vi "Select HDF5 Dialog Core.vi"(0 "Initial File Path":path, 1 "Close HDF5 File?":bool, 2 "Item Filters":T4 {"Object Types (any)" items=["H5G_UNKNOWN"=-1, "H5G_GROUP"=0, "H5G_DATASET"=1, "H5G_TYPE"=2, "H5G_LINK"=3, "H5G_UDLINK"=4]}, 3 "File Browse Options":T7, 5 "HDF5 File Ref":T9, 7 "Initial Object Path":string, 9 "Path visible":bool=TRUE, 11 "error in":errorcluster, 12 "Operation Modes":cluster{"File":T1, "Object":T2}={"File"=enum."open or create", "Object"=enum."open or create"}, 13 "Window":T6={"Behavior"=enum."Modal", "Position"={"Left"=0, "Top"=0, "Right"=600, "Bottom"=400}, "Center"=TRUE, "Title"="Select an HDF5 Object"}) -> (4 "File Path out":path, 6 "HDF5 File Ref out":T9, 8 "Object Path out":string, 10 "OK?":bool, 14 "Object operation out":T8(ring), 15 "error out":errorcluster)   [LabVIEW 2017]
uses:
  <vilib>/UPVI/lvhdf5/library.llb/HDF5 Ref.ctl
  <vilib>/Utility/miscctls.llb/LVRectTypeDef.ctl
  <vilib>/UPVI/lvhdf5/group.llb/H5G_obj_t.ctl
  <vilib>/UPVI/lvhdf5/file.llb/LVH5F Operation.ctl
  <vilib>/UPVI/lvhdf5/dataset.llb/LVH5D Operation.ctl
  <vilib>/UPVI/lvhdf5/utility.llb/private/TreeIconsEnum.ctl
  <vilib>/UPVI/lvhdf5/object.llb/H5O_type_t.ctl
  <vilib>/UPVI/lvhdf5/identifier.llb/H5Iget_type.vi
panel:
  in  "File Path":path
  in  "Object Path":string
  in  "Cancel Button":bool
  in  "OK Button":bool
  in  "Attributes":i32(listbox)
  in  "Hierarchy":string(tree)
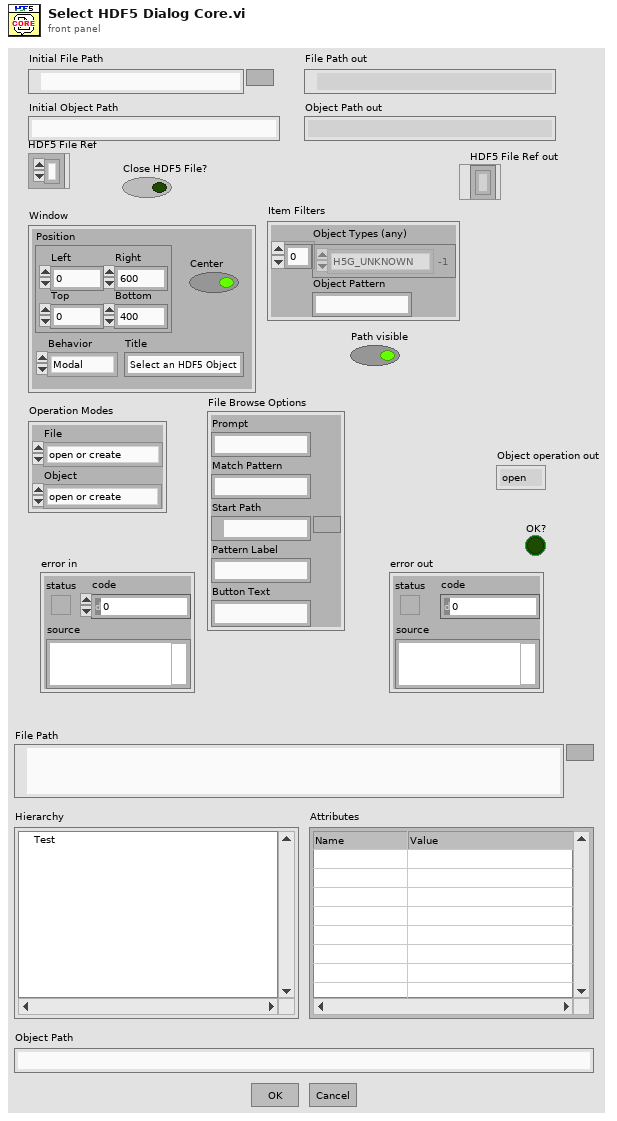
[diagram p1: front panel]
types:
  T1 = typedef "LVH5F Operation.ctl" = enum16{"open", "open or create", "create or replace", "create or replace (with confirmation)", "create", "open (read only)"}
  T2 = typedef "LVH5D Operation.ctl" = enum16{"open", "replace", "create", "open or create", "create or replace", "create or replace with confirmation"}
  T3 = typedef "H5G_obj_t.ctl" = i32
  T4 = cluster{"Object Types (any)":T3[], "Object Pattern":string}
  T5 = typedef "LVRectTypeDef.ctl" = cluster{"Left":i16, "Top":i16, "Right":i16, "Bottom":i16}
  T6 = cluster{"Behavior":enum32{"Invalid", "Default", "Floating", "Floating/Auto-Hide", "Modal"}, "Position":T5, "Center":bool, "Title":string}
  T7 = cluster{"Prompt":string, "Match Pattern":string, "Start Path":path, "Pattern Label":string, "Button Text":string}
  T8 = enum16{"open", "replace", "create", "open or create", "replace or create", "replace or create with confirmation"}
  T9 = typedef "HDF5 Ref.ctl" = refnum<k1>
  T10 = cluster{"File Path":refnum<vi>, "Hierarchy":refnum<vi>, "Attributes":refnum<vi>, "Object Path":refnum<vi>, "OK Button":refnum<vi>, "Cancel Button":refnum<vi>}
  T11 = enum32{"existing file", "new file", "new or existing file", "existing dir", "new dir", "new or existing dir", "existing file (use LLBs)", "new file (use LLBs)", "new or existing file (use LLBs)", "new or existing file or directory (use LLBs)", "existing dir (use LLBs)", "new dir (use LLBs)", "new or existing dir (use LLBs)", "existing file or dir", "new file or dir", "new or existing file or dir", "existing file or dir (use LLBs)", "new file or dir (use LLBs)"}
  T12 = enum8{"Enabled", "Disabled", "Disabled and Grayed Out"}
  T13 = typedef "TreeIconsEnum.ctl" = enum16{"None", "Closed Group", "Open Group", "Array Dataset", "Compound Dataset", "Datatype"}
  T14 = enum16{"open", "create", "replace", "cancel", "error"}
  T15 = enum32{"Invalid", "Default", "Floating", "Floating/Auto-Hide", "Modal"}
  T16 = cluster{"Prompt":string, "Match Pattern":string, "Mode":enum32{"existing file", "new file", "new or existing file", "existing dir", "new dir", "new or existing dir", "existing file (use LLBs)", "new file (use LLBs)", "new or existing file (use LLBs)", "new or existing file or directory (use LLBs)", "existing dir (use LLBs)", "new dir (use LLBs)", "new or existing dir (use LLBs)", "existing file or dir", "new file or dir", "new or existing file or dir", "existing file or dir (use LLBs)", "new file or dir (use LLBs)"}, "Start Path":path, "Pattern Label":string, "Button Text":string}
  T17 = enum16{"Left Button", "Center Button", "Right Button", "Window Close"}
  T18 = typedef "H5O_type_t.ctl" = i32
  T19 = typedef "LVH5O_info_t.ctl" = cluster{"fileno":u32, "addr":u64, "type":T18, "rc":u32, "atime":timestamp, "mtime":timestamp, "ctime":timestamp, "btime":timestamp, "num_attrs":i64, "H5O_hdr_info_t":T20, "meta_size":cluster{"obj":T21, "attr":T21}}
  T20 = typedef "H5O_hdr_info_t.ctl" = cluster{"version":u32, "nmesgs":u32, "nchuncks":u32, "flags":u32, "space":cluster{"total":u64, "meta":u64, "mesg":u64, "free":u64}, "mesg":cluster{"present":u64, "shared":u64}}
  T21 = typedef "H5_ih_info_t.ctl" = cluster{"index_size":u64, "heap_size":u64}
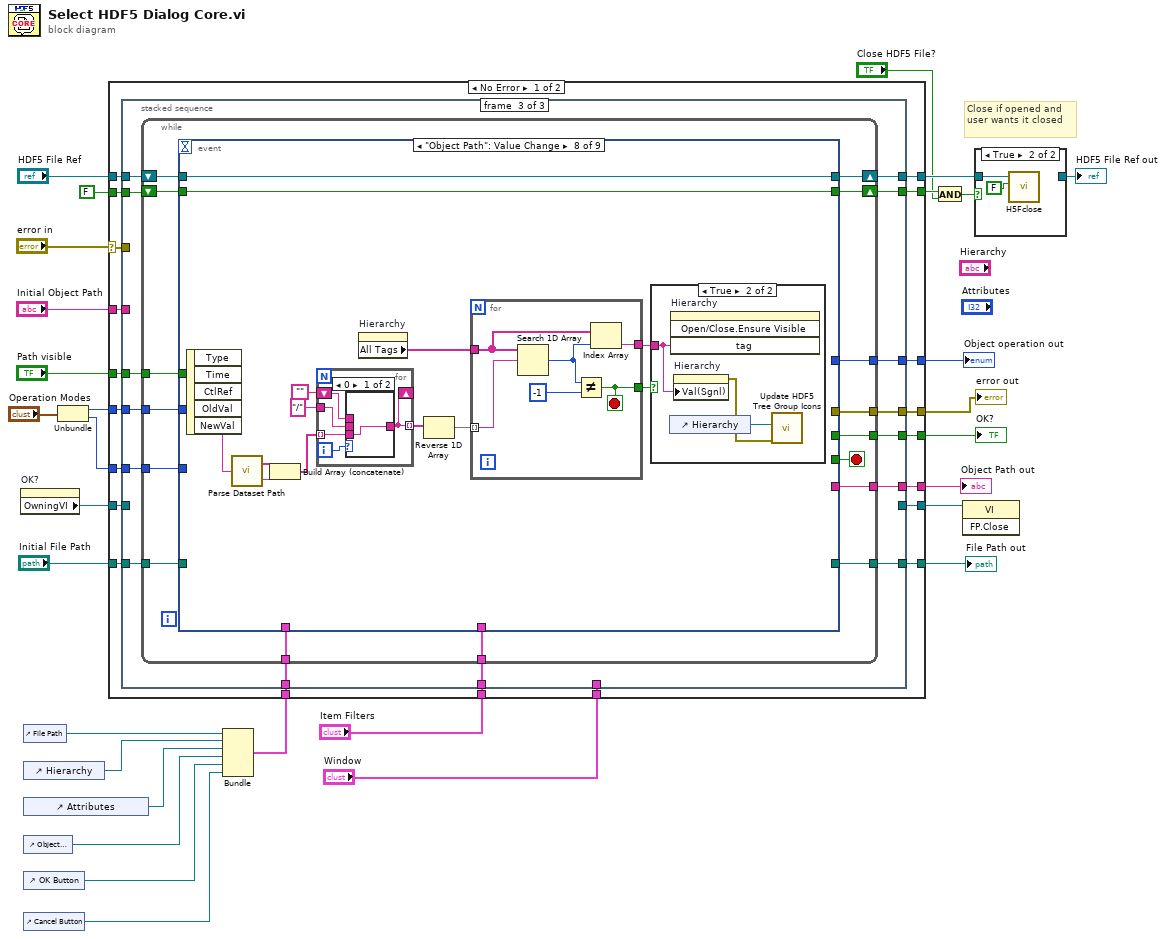
[diagram p0: block diagram]
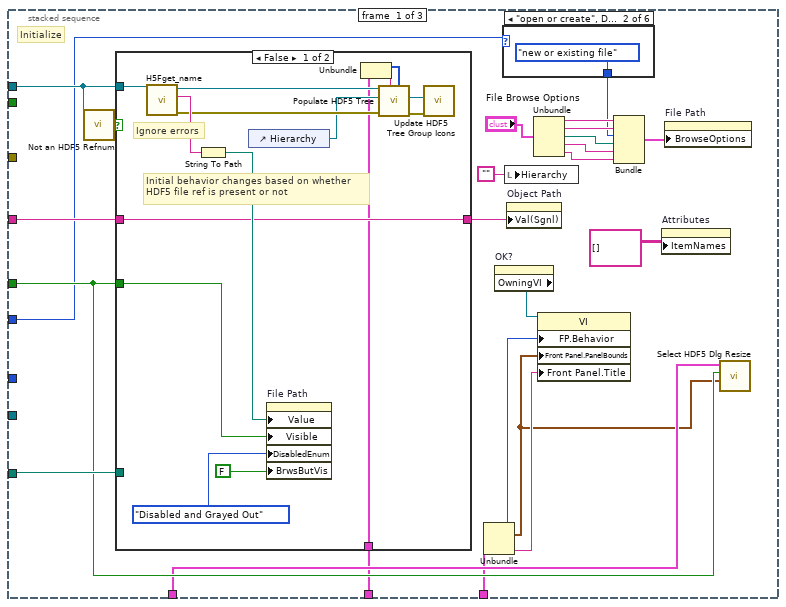
[diagram p2: hidden frame]
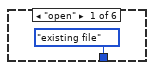
[diagram p3: hidden frame]
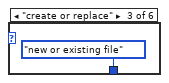
[diagram p4: hidden frame]
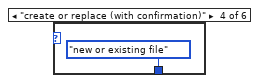
[diagram p5: hidden frame]
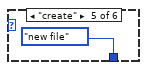
[diagram p6: hidden frame]
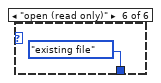
[diagram p7: hidden frame]
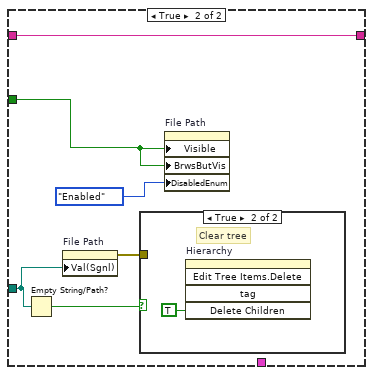
[diagram p8: hidden frame]
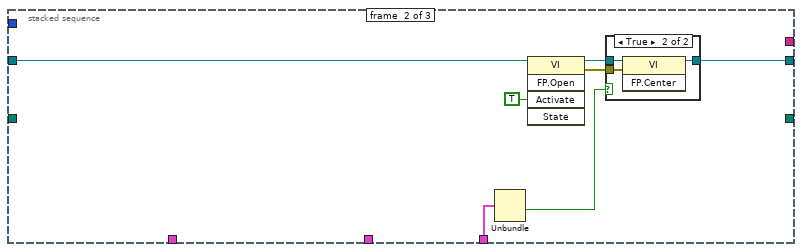
[diagram p10: hidden frame]
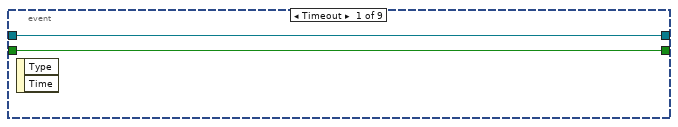
[diagram p12: hidden frame]
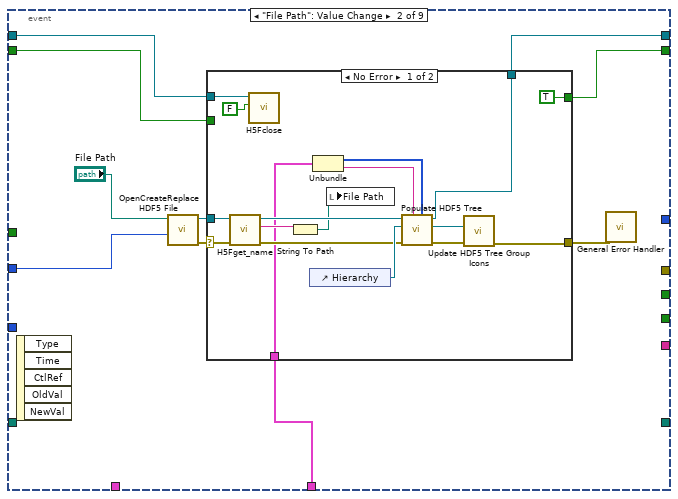
[diagram p13: hidden frame]
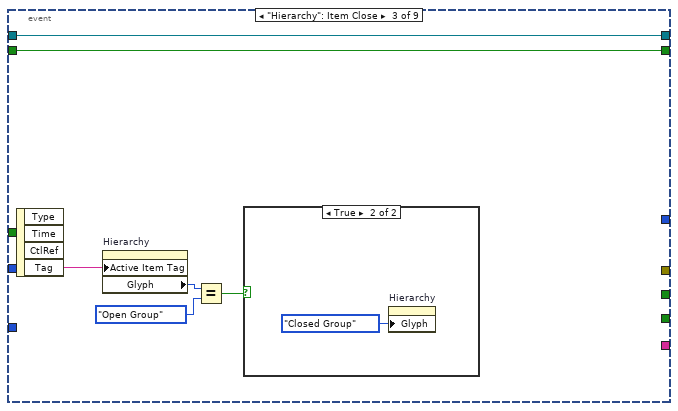
[diagram p15: hidden frame]
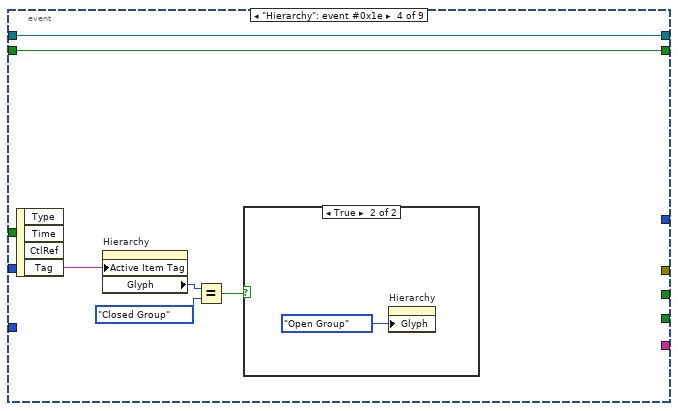
[diagram p17: hidden frame]
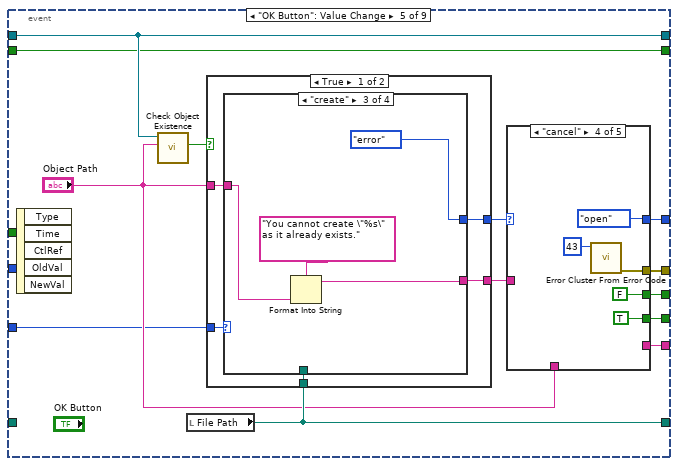
[diagram p19: hidden frame]
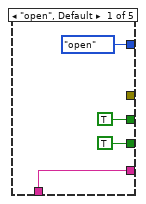
[diagram p20: hidden frame]
diagram:
  # "Close if opened and user wants it closed"
  n1 = property on="OK?" class="Bool (strict)"() -> ("OwningVI"=w1:refnum<vi>)  [unwired: 2 in, 2 out]
  n2 = control-ref of="File Path"() -> (w14:refnum<vi>)
  n3 = control-ref of="Hierarchy"() -> (w15:refnum<vi>)
  n4 = control-ref of="Attributes"() -> (w16:refnum<vi>)
  n5 = control-ref of="Object Path"() -> (w17:refnum<vi>)
  n6 = control-ref of="OK Button"() -> (w18:refnum<vi>)
  n7 = control-ref of="Cancel Button"() -> (w19:refnum<vi>)
  n8 = Unbundle("Operation Modes") -> ("File"=w4:T1, "Object"=w5:T2)
  n9 = Bundle("File Path"=w14, "Hierarchy"=w15, "Attributes"=w16, "Object Path"=w17, "OK Button"=w18, "Cancel Button"=w19) -> (w13:T10)  [unwired: 1 in]
  n10 = case shown="No Error" "error in" {
    selector: "error in" -> [w42 w341]
    tunnel: [w50 w342] -> w30
    tunnel: [w49 w339] -> w28
    tunnel: [w48 FALSE] -> w27
    tunnel: [w47 _] -> w26
    tunnel: "Initial File Path" -> [w46 w339]
    tunnel: [w45 w341] -> w24
    tunnel: "HDF5 File Ref" -> [w44 w342]
    tunnel: "Path visible" -> [w43 _]
    tunnel: [w41 _] -> w20
    tunnel: w13 -> [w40 _]
    tunnel: FALSE -> [w39 _]
    tunnel: [w38 FALSE] -> w11
    tunnel: "Initial Object Path" -> [w37 _]
    tunnel: "Item Filters" -> [w36 _]
    tunnel: w5 -> [w35 _]
    tunnel: w4 -> [w34 _]
    tunnel: "Window" -> [w33 _]
    tunnel: [w32 w337] -> w2
    tunnel: w1 -> [w31 w337]
    frame No Error {
      n11 = stacked-sequence {
        tunnel: [_ _ w128] -> w50
        tunnel: [_ _ w127] -> w49
        tunnel: [_ _ w126] -> w48
        tunnel: [_ _ w125] -> w47
        tunnel: w46 -> [w72 _ w124]
        tunnel: [_ _ w123] -> w45
        tunnel: w44 -> [w73 _ w122]
        tunnel: w43 -> [w70 _ w119]
        tunnel: w42 -> [_ _ _]
        tunnel: [_ _ w121] -> w41
        tunnel: w40 -> [w69 _ w120]
        tunnel: w39 -> [_ _ w118]
        tunnel: [_ _ w117] -> w38
        tunnel: w37 -> [w68 _ _]
        tunnel: w36 -> [w66 _ w116]
        tunnel: w35 -> [_ _ w115]
        tunnel: w34 -> [w54 _ w114]
        tunnel: w33 -> [w65 w104 _]
        tunnel: [_ w105 _] -> w32
        tunnel: w31 -> [_ w108 _]
        frame #0 {
          # "Initialize"
          n12 = call <vilib>:"Not an HDF5 Refnum.vi"("HDF5 Ref"=w73) -> ("Not an HDF5 Refnum"=w74:bool)
          n13 = case shown="False" w74 {
            tunnel: w73 -> [w94 _]
            tunnel: w72 -> [_ w97]
            tunnel: w70 -> [w91 w99]
            tunnel: w68 -> [w89 w98]
            tunnel: [w89 w98] -> w67
            tunnel: w66 -> [w85 _]
            frame False {
              # "Initial behavior changes based on whether\nHDF5 file ref is present or not"
              # "Ignore errors"
              n14 = call <vilib>:"H5Fget_name.vi"("HDF5 Attr Ref"=w94) -> ("error out"=w87:errorcluster, "Name"=w95:string, "HDF5 Attr Ref out"=w88:T9)  [unwired: 6 in]
              n15 = String To Path(string=w95) -> (path=w90:path)
              n16 = control-ref of="Hierarchy"() -> (w86:refnum<vi>)
              n17 = property on="File Path" class="Path"("Value"=w90, "Visible"=w91, "DisabledEnum"=T12."Disabled and Grayed Out" ("Disabled"), "BrwsButVis"=FALSE ("Browse Button:Visible")) -> ()  [unwired: 2 in, 2 out]
              n18 = Unbundle(w85) -> ("Object Types (any)"=w84:T3[], "Object Pattern"=w83:string)
              n19 = call <vilib>:"Populate HDF5 Tree.vi"("Object Types (any)"=w84, "pattern"=w83, "error in"=w87, "Tree"=w86, "HDF5 Ref"=w88) -> ("error out"=w82:errorcluster, "Tree out"=w81:refnum<vi>)  [unwired: 4 in, 1 out]
              n20 = call <vilib>:"Update HDF5 Tree Group Icons.vi"("error in"=w82, "Tree"=w81) -> ()  [unwired: 8 in, 2 out]
            }
            frame True {
              n21 = Empty String/Path?(string/path=w97) -> (empty?=w101:bool)
              n22 = property on="File Path" class="Path"("Val(Sgnl)"=w97) -> (error out=w96:errorcluster)  [unwired: 2 in, 1 out]
              n23 = case shown="True" w101 {
                tunnel: w96 -> [_ _]
                frame False {
                }
                frame True {
                  # "Clear tree"
                  n24 = invoke on="Hierarchy" class="Tree (strict)" method="Edit Tree Items.Delete"("Delete Children"=TRUE ("Delete Children?")) -> ()  [unwired: 4 in, 5 out]
                }
              }
              n25 = property on="File Path" class="Path"("Visible"=w99, "BrwsButVis"=w99, "DisabledEnum"=T12."Enabled" ("Disabled")) -> ()  [unwired: 2 in, 2 out]
            }
          }
          n26 = Unbundle(w65) -> ("Behavior"=w64:T15, "Position"=w62:T5, "Title"=w63:string)  [unwired: 1 out]
          n27 = property on="OK?" class="Bool (strict)"() -> ("OwningVI"=w71:refnum<vi>)  [unwired: 2 in, 2 out]
          n28 = case shown="\"open or create\", Default" w54 {
            tunnel: [T11."existing file" ("Mode") T11."new or existing file" ("Mode") T11."new or existing file" ("Mode") T11."new or existing file" ("Mode") T11."new file" ("Mode") T11."existing file" ("Mode")] -> w53
            frame "open" {
            }
            frame "open or create", Default {
            }
            frame "create or replace" {
            }
            frame "create or replace (with confirmation)" {
            }
            frame "create" {
            }
            frame "open (read only)" {
            }
          }
          n29 = local write "Hierarchy"("") -> ()
          n30 = property on="Object Path" class="Str"("Val(Sgnl)"=w67) -> ()  [unwired: 2 in, 2 out]
          n31 = Unbundle("File Browse Options") -> ("Prompt"=w59:string, "Match Pattern"=w58:string, "Start Path"=w57:path, "Pattern Label"=w56:string, "Button Text"=w55:string)
          n32 = property class="VI"(reference=w71, "FP.Behavior"=w64, "Front Panel.PanelBounds"=w62, "Front Panel.Title"=w63) -> ()  [unwired: 1 in, 2 out]
          n33 = Bundle("Prompt"=w59, "Match Pattern"=w58, "Mode"=w53, "Start Path"=w57, "Pattern Label"=w56, "Button Text"=w55) -> (w52:T16)  [unwired: 1 in]
          n34 = property on="Attributes" class="MCListbox (strict)"("ItemNames"=string[][] [] ("Item Names")) -> ()  [unwired: 2 in, 2 out]
          n35 = property on="File Path" class="Path"("BrowseOptions"=w52) -> ()  [unwired: 2 in, 2 out]
          n36 = call <vilib>:"Select HDF5 Dlg Resize.vi"("NewBnds"=w62, "Display Path?"=w70, "Select HDF5 Dlg Items"=w69) -> ()  [unwired: 8 in, 1 out]
        }
        frame #1 {
          n37 = Unbundle(w104) -> ("Center"=w103:bool)  [unwired: 3 out]
          n38 = invoke class="VI" method="FP.Open"(reference=w108, "Activate"=TRUE ("Activate?")) -> (reference out=w107:refnum<vi>, error out=w106:errorcluster)  [unwired: 3 in, 3 out]
          n39 = case shown="True" w103 {
            tunnel: w107 -> [w110 w113]
            tunnel: w106 -> [_ w112]
            tunnel: [w110 w111] -> w105
            frame False {
            }
            frame True {
              n40 = invoke class="VI" method="FP.Center"(reference=w113, error in=w112) -> (reference out=w111:refnum<vi>)  [unwired: 1 in, 2 out]
            }
          }
        }
        frame #2 {
          n41 = while {
            shift-right: [w144] -> w128
            shift-left: w122 -> [w143]
            tunnel: [w142] -> w127
            tunnel: [w141] -> w123
            tunnel: [w139] -> w126
            tunnel: [w138] -> w125
            tunnel: w124 -> [w137]
            tunnel: [w136] -> w121
            tunnel: w120 -> [w135]
            tunnel: w119 -> [w134]
            shift-right: [w133] -> w117
            shift-left: w118 -> [w132]
            tunnel: w116 -> [w131]
            tunnel: w115 -> [w130]
            tunnel: w114 -> [w129]
            stop <- w140 stop-if-true
            n42 = event shown="[7] \"Object Path\": Value Change" {
              selector: _ -> [_ _ _ _ _ _ _ _ _]
              dyn-events: _ -> [_ _ _ _ _ _ _ _ _]
              timeout: _ -> [_ _ _ _ _ _ _ _ _]
              tunnel: [w146 w156 w178 w185 w203 w258 w272 w312 w336] -> w144
              tunnel: w143 -> [w146 w151 w178 w185 w203 w258 w272 w312 w336]
              tunnel: [_ _ _ _ w202 w261 _ _ _] -> w142
              tunnel: [_ _ _ _ w197 w259 _ _ _] -> w141
              tunnel: [_ _ _ _ w198 TRUE _ _ _] -> w140
              tunnel: [_ _ _ _ w196 FALSE _ _ _] -> w139
              tunnel: [_ _ _ _ w195 _ _ _ _] -> w138
              tunnel: w137 -> [_ _ _ _ _ w261 _ _ _]
              tunnel: [_ _ _ _ w193 _ _ _ _] -> w136
              tunnel: w135 -> [_ _ _ _ _ _ _ _ w333]
              tunnel: w134 -> [_ _ _ _ _ _ _ _ w334]
              tunnel: [w145 w150 w177 w184 w192 w256 w263 w305 w332] -> w133
              tunnel: w132 -> [w145 w149 w177 w184 w192 w256 w263 w305 w332]
              tunnel: w131 -> [_ w148 _ _ _ _ _ _ _]
              tunnel: w130 -> [_ _ _ _ w191 _ _ _ _]
              tunnel: w129 -> [_ w147 _ _ _ _ _ _ _]
              event Timeout {
                n43 = event-data() -> ()  [unwired: 1 in, 2 out]
              }
              event "File Path": Value Change {
                n44 = event-data() -> ()  [unwired: 1 in, 5 out]
                n45 = call <vilib>:"OpenCreateReplace HDF5 File.vi"("function (open or create)"=w147, "path"="File Path") -> ("error out"=w153:errorcluster, "HDF5 Ref out"=w155:T9)  [unwired: 6 in]
                n46 = case shown="No Error" w153 {
                  selector: w153 -> [w166 w175]
                  tunnel: [w172 w176] -> w156
                  tunnel: w155 -> [w171 _]
                  tunnel: [w158 w175] -> w152
                  tunnel: w151 -> [w165 w176]
                  tunnel: [TRUE w174] -> w150
                  tunnel: w149 -> [_ w174]
                  tunnel: w148 -> [w162 _]
                  frame No Error {
                    n47 = call <vilib>:"H5Fget_name.vi"("error in (no error)"=w166, "HDF5 Attr Ref"=w171) -> ("error out"=w170:errorcluster, "Name"=w168:string, "HDF5 Attr Ref out"=w169:T9)  [unwired: 5 in]
                    n48 = call <vilib>:"H5Fclose.vi"("Close All Open Objects (T)"=FALSE, "HDF5 Ref"=w165) -> ()  [unwired: 7 in, 1 out]
                    n49 = String To Path(string=w168) -> (path=w167:path)
                    n50 = control-ref of="Hierarchy"() -> (w173:refnum<vi>)
                    n51 = Unbundle(w162) -> ("Object Types (any)"=w161:T3[], "Object Pattern"=w160:string)
                    n52 = local write "File Path"(w167) -> ()
                    n53 = call <vilib>:"Populate HDF5 Tree.vi"("Object Types (any)"=w161, "pattern"=w160, "error in"=w170, "Tree"=w173, "HDF5 Ref"=w169) -> ("error out"=w159:errorcluster, "Tree out"=w157:refnum<vi>, "HDF5 Ref out"=w172:T9)  [unwired: 4 in]
                    n54 = call <vilib>:"Update HDF5 Tree Group Icons.vi"("error in"=w159, "Tree"=w157) -> ("error out"=w158:errorcluster)  [unwired: 8 in, 1 out]
                  }
                  frame Error {
                  }
                }
                n55 = call <vilib>:"General Error Handler.vi"("error in (no error)"=w152) -> ()  [unwired: 10 in, 5 out]
              }
              event "Hierarchy": Item Close {
                n56 = event-data() -> ("Tag"=w180:string)  [unwired: 1 in, 3 out]
                n57 = property on="Hierarchy" class="Tree (strict)"("Active Item Tag"=w180) -> ("Glyph"=w182:i32)  [unwired: 2 in, 2 out]
                n58 = Equal?(x=w182, y=TreeIconsEnum."Open Group" ("TreeIcons")) -> (x = y?=w179:bool)
                n59 = case shown="True" w179 {
                  frame False {
                  }
                  frame True {
                    n60 = property on="Hierarchy" class="Tree (strict)"("Glyph"=TreeIconsEnum."Closed Group" ("TreeIcons")) -> ()  [unwired: 2 in, 2 out]
                  }
                }
              }
              event "Hierarchy": event #0x1e {
                n61 = event-data() -> ("Tag"=w187:string)  [unwired: 1 in, 3 out]
                n62 = property on="Hierarchy" class="Tree (strict)"("Active Item Tag"=w187) -> ("Glyph"=w189:i32)  [unwired: 2 in, 2 out]
                n63 = Equal?(x=w189, y=TreeIconsEnum."Closed Group" ("TreeIcons")) -> (x = y?=w186:bool)
                n64 = case shown="True" w186 {
                  frame False {
                  }
                  frame True {
                    n65 = property on="Hierarchy" class="Tree (strict)"("Glyph"=TreeIconsEnum."Open Group" ("TreeIcons")) -> ()  [unwired: 2 in, 2 out]
                  }
                }
              }
              event "OK Button": Value Change {
                n66 = event-data() -> ()  [unwired: 1 in, 5 out]
                n67 = call <vilib>:"Check Object Existence.vi"("name"="Object Path", "HDF5 Ref"=w203) -> ("Exists"=w201:bool)  [unwired: 5 in, 2 out]
                n68 = local read "File Path"() -> (w202:path)
                n69 = case shown="True" w201 {
                  tunnel: [w226 w250] -> w199
                  tunnel: "Object Path" -> [w229 w249]
                  tunnel: w202 -> [w228 w248]
                  tunnel: [w227 w247] -> w200
                  tunnel: w191 -> [w225 w246]
                  frame True {
                    n70 = case shown="\"create\"" w225 {
                      tunnel: [_ _ w232 _] -> w226
                      tunnel: w229 -> [_ _ w234 w236]
                      tunnel: w228 -> [_ _ _ _]
                      tunnel: [T14."open" T14."replace" T14."error" w237] -> w227
                      frame "open", "open or create", Default {
                      }
                      frame "replace", "create or replace" {
                      }
                      frame "create" {
                        n71 = Format Into String(format string="You cannot create \"%s\" as it already exists." ("error message (\"\")"), w234) -> (resulting string=w232:string)  [unwired: 2 in, 1 out]
                      }
                      frame "create or replace with confirmation" {
                        n72 = Format Into String(format string="\"%s\" exists.\\nWould you like to open it or replace it?", w236) -> (resulting string=w241:string)  [unwired: 2 in, 1 out]
                        n73 = call <vilib>:"Three Button Dialog.vi"("Center Button Text (\"No\")"="Replace" ("Center Button Text (\"No\")"), "Left Button Text (\"Yes\")"="Open" ("Left Button Text (\"Yes\")"), "message"=w241) -> ("Which Button?"=w238:T17)  [unwired: 8 in]
                        n74 = case shown="\"Center Button\"" w238 {
                          tunnel: [T14."open" T14."replace" T14."cancel"] -> w237
                          frame "Left Button", Default {
                          }
                          frame "Center Button" {
                          }
                          frame "Right Button" {
                          }
                        }
                      }
                    }
                  }
                  frame False {
                    n75 = case shown="\"open\", \"replace\", Default" w246 {
                      tunnel: [w251 _] -> w250
                      tunnel: w249 -> [w252 _]
                      tunnel: w248 -> [_ _]
                      tunnel: [T14."error" T14."create"] -> w247
                      frame "open", "replace", Default {
                        n76 = Format Into String(format string="\"%s\" not found." ("error message (\"\")"), w252) -> (resulting string=w251:string)  [unwired: 2 in, 1 out]
                      }
                      frame "create".."create or replace with confirmation" {
                      }
                    }
                  }
                }
                n77 = case shown="\"cancel\"" w200 {
                  tunnel: w199 -> [_ _ _ _ w222]
                  tunnel: [TRUE TRUE TRUE TRUE FALSE] -> w198
                  tunnel: [_ _ _ w220 _] -> w197
                  tunnel: [TRUE TRUE TRUE FALSE FALSE] -> w196
                  tunnel: [w205 w209 w213 _ _] -> w195
                  tunnel: "Object Path" -> [w205 w209 w213 _ _]
                  tunnel: [T8."open" ("Object operation 2") T8."create" ("Object operation 2") T8."replace" ("Object operation 2") T8."open" ("Object operation 2") T8."open" ("Object operation 2")] -> w193
                  frame "open", Default {
                  }
                  frame "create" {
                  }
                  frame "replace" {
                  }
                  frame "cancel" {
                    n78 = call <vilib>:"Error Cluster From Error Code.vi"("error code (0)"=43) -> ("error out"=w220:errorcluster)  [unwired: 8 in]
                  }
                  frame "error" {
                    n79 = One Button Dialog(message=w222) -> ()  [unwired: 1 in, 1 out]
                  }
                }
              }
              event "Cancel Button": Value Change {
                n80 = event-data() -> ()  [unwired: 1 in, 5 out]
                n81 = call <vilib>:"Error Cluster From Error Code.vi"("error code (0)"=43) -> ("error out"=w259:errorcluster)  [unwired: 8 in]
              }
              event "Hierarchy": Value Change {
                (unwired) T18 0 items=["H5O_TYPE_UNKNOWN"=-1, "H5O_TYPE_GROUP"=0, "H5O_TYPE_DATASET"=1, "H5O_TYPE_NAMED_DATATYPE"=2] ("type")
                n82 = event-data() -> ("NewVal"=w264:string)  [unwired: 1 in, 4 out]
                n83 = call <vilib>:"H5Oget_info_by_name.vi"("Name"=w264, "HDF5 Ref"=w272) -> ("error out"=w269:errorcluster, "Object Info"=w271:T19, "HDF5 Ref out"=w268:T9)  [unwired: 5 in]
                n84 = Unbundle By Name(w271) -> ("type"=w270:T18)
                n85 = case shown="2" w270 {
                  tunnel: w269 -> [w285 w291 w296 _]
                  tunnel: w268 -> [w286 w292 w298 _]
                  tunnel: w264 -> [w284 w290 w297 _]
                  tunnel: [w282 w289 w295 _] -> w266
                  tunnel: [w281 w288 w294 _] -> w267
                  tunnel: [TRUE TRUE TRUE FALSE] -> w265
                  frame 0 {
                    # "GROUP"
                    n86 = call <vilib>:"H5Gopen.vi"("error in (no error)"=w285, "Name"=w284, "HDF5 Ref"=w286) -> ("error out"=w281:errorcluster, "HDF5 Group Ref"=w282:T9)  [unwired: 4 in, 1 out]
                  }
                  frame 1 {
                    # "DATASET"
                    n87 = call <vilib>:"H5Dopen.vi"("error in (no error)"=w291, "name"=w290, "HDF5 Ref"=w292) -> ("error out"=w288:errorcluster, "HDF5 Dataset Ref"=w289:T9)  [unwired: 4 in, 1 out]
                  }
                  frame 2 {
                    # "DATATYPE"
                    n88 = call <vilib>:"H5Topen.vi"("error in (no error)"=w296, "name"=w297, "HDF5 Location"=w298) -> ("error out"=w294:errorcluster, "HDF5 Type Ref"=w295:T9)  [unwired: 4 in, 1 out]
                  }
                  frame -1, Default {
                  }
                }
                n89 = local write "Object Path"(w264) -> ()
                n90 = case shown="True" w265 {
                  tunnel: w267 -> [_ w280]
                  tunnel: w266 -> [_ w279]
                  frame False {
                    n91 = property on="Attributes" class="MCListbox (strict)"("ItemNames"=string[][] [] ("Item Names")) -> ()  [unwired: 2 in, 2 out]
                  }
                  frame True {
                    n92 = call <vilib>:"Read All Attributes.vi"("error in (no error)"=w280, "HDF5 Ref"=w279) -> ("error out"=w274:errorcluster, "Values"=w277:variant[], "Names"=w278:string[], "HDF5 Ref out"=w275:T9)  [unwired: 4 in]
                    n93 = call <vilib>:"Format Attributes as Table.vi"("Values"=w277, "Names"=w278) -> ("Formatted Table"=w276:string[][])  [unwired: 8 in, 1 out]
                    n94 = call <vilib>:"H5Idec_ref.vi"("error in (no error)"=w274, "HDF5 Ref"=w275) -> ()  [unwired: 5 in, 3 out]
                    n95 = property on="Attributes" class="MCListbox (strict)"("ItemNames"=w276) -> ()  [unwired: 2 in, 2 out]
                  }
                }
              }
              event "Object Path": Value Change {
                n96 = event-data() -> ("NewVal"=w303:string)  [unwired: 1 in, 4 out]
                n97 = call <vilib>:"Parse Dataset Path.vi"("Dataset path"=w303) -> ("Groups"=w302:string[], "Dataset"=w301:string)
                n98 = Build Array (concatenate)(w302, w301) -> (w300:string[])
                n99 = for {
                  tunnel: w300 -> [w326] mode=indexing
                  shift-right: [w323] -> _
                  shift-left: "" -> [w324]
                  tunnel: "/" ("delimiter (Tab)") -> [w325]
                  tunnel: [w323] -> w310 mode=indexing
                  i -> [w322]
                  n100 = case shown="0" w322 {
                    tunnel: w326 -> [w327 w331]
                    tunnel: w325 -> [_ w330]
                    tunnel: w324 -> [_ w329]
                    tunnel: [w327 w328] -> w323
                    frame 0 {
                    }
                    frame 1, Default {
                      n101 = Concatenate Strings(w329, w330, w331) -> (w328:string)
                    }
                  }
                }
                n102 = property on="Hierarchy" class="Tree (strict)"() -> ("All Tags"=w309:string[])  [unwired: 2 in, 2 out]
                n103 = Reverse 1D Array(array=w310) -> (reversed array=w308:string[])
                n104 = for {
                  tunnel: w309 -> [w318]
                  tunnel: w308 -> [w321] mode=indexing
                  tunnel: [w317] -> w307
                  tunnel: [w316] -> w306
                  stop <- w316 stop-if-true
                  n105 = Search 1D Array(1D array=w318, element=w321) -> (index of element=w319:i32)  [unwired: 1 in]
                  n106 = Not Equal?(x=w319, y=-1) -> (x != y?=w316:bool)
                  n107 = Index Array(array=w318, index=w319) -> (element=w317:string)
                }
                n108 = case shown="True" w306 {
                  tunnel: w307 -> [_ w315]
                  frame False {
                  }
                  frame True {
                    n109 = control-ref of="Hierarchy"() -> (w313:refnum<vi>)
                    n110 = invoke on="Hierarchy" class="Tree (strict)" method="Open/Close.Ensure Visible"("tag"=w315) -> ()  [unwired: 3 in, 4 out]
                    n111 = property on="Hierarchy" class="Tree (strict)"("Val(Sgnl)"=w315) -> (error out=w314:errorcluster)  [unwired: 2 in, 1 out]
                    n112 = call <vilib>:"Update HDF5 Tree Group Icons.vi"("error in"=w314, "Tree"=w313) -> ()  [unwired: 8 in, 2 out]
                  }
                }
              }
              event Panel Resize {
                n113 = event-data() -> ("NewBnds"=w335:T5)  [unwired: 1 in, 6 out]
                n114 = call <vilib>:"Select HDF5 Dlg Resize.vi"("NewBnds"=w335, "Display Path?"=w334, "Select HDF5 Dlg Items"=w333) -> ()  [unwired: 8 in, 1 out]
              }
            }
          }
        }
      }
    }
    frame Error {
    }
  }
  "File Path out" <- w28
  "OK?" <- w27
  "Object Path out" <- w26
  "error out" <- w24
  "Object operation out" <- w20
  n115 = And(x=w11, y="Close HDF5 File?") -> (x .and. y?=w9:bool)
  n116 = invoke class="VI" method="FP.Close"(reference=w2) -> ()  [unwired: 2 in, 3 out]
  n117 = case shown="True" w9 {
    tunnel: w30 -> [w343 w345]
    tunnel: [w343 _] -> w29
    frame False {
    }
    frame True {
      n118 = call <vilib>:"H5Fclose.vi"("Close All Open Objects (T)"=FALSE, "HDF5 Ref"=w345) -> ()  [unwired: 7 in, 1 out]
    }
  }
  "HDF5 File Ref out" <- w29
